vi "Pololu-Convert Degrees to Encoder Units.vi"(4 "Deg Max":u16=180, 5 "Encoder Units Max":u16, 6 "Deg Min":u16, 7 "Encoder Units Min":u16, 8 "Error In":errorcluster, 11 "Position Deg":u16) -> (0 "Error Out":errorcluster, 3 "Position Encoder Units":u16)   [LabVIEW 2018]
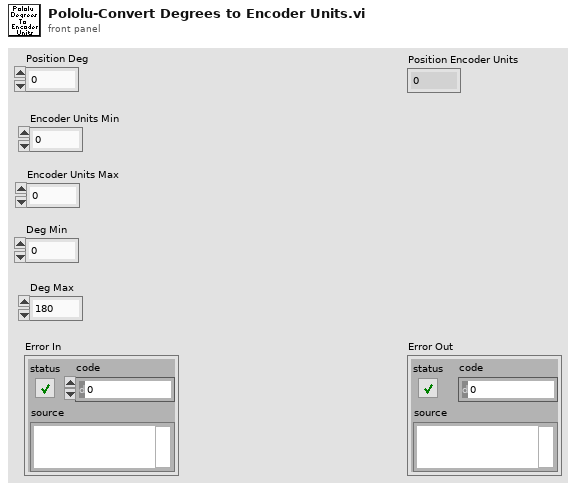
[diagram p1: front panel]
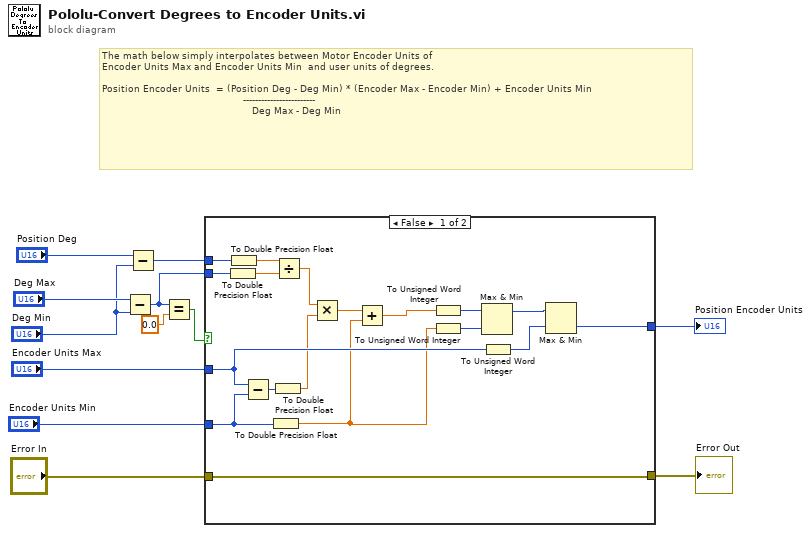
[diagram p0: block diagram]
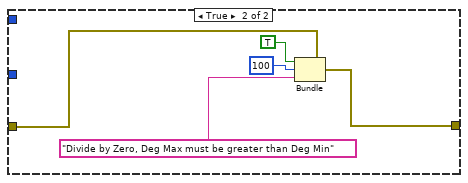
[diagram p2: hidden frame]
diagram:
  # "The math below simply interpolates between Motor Encoder Units of \nEncoder Units Max and Encoder Units Min  and user units of degrees.\n\nPosition Encoder Units  = (Position Deg - Deg Min) * (Encoder Max - Encoder Min) + Encoder Units Min\n                                               ------------------------\n                                                  Deg Max - Deg Min"
  n1 = Subtract(x="Deg Max", y="Deg Min") -> (x-y=w4:u16)
  n2 = Subtract(x="Position Deg", y="Deg Min") -> (x-y=w11:u16)
  n3 = Equal?(x=w4, y=0.0) -> (x = y?=w5:bool)
  n4 = case shown="False" w5 {
    tunnel: [w28 _] -> w12
    tunnel: w11 -> [w20 _]
    tunnel: "Encoder Units Max" -> [w24 _]
    tunnel: "Encoder Units Min" -> [w14 _]
    tunnel: w4 -> [w19 _]
    tunnel: [w21 w31] -> w3
    tunnel: "Error In" -> [w21 w35]
    frame False {
      n5 = To Double Precision Float(number=w19) -> (double precision float=w17:dbl)
      n6 = To Double Precision Float(number=w20) -> (double precision float=w18:dbl)
      n7 = Subtract(x=w24, y=w14) -> (x-y=w16:u16)
      n8 = To Double Precision Float(number=w14) -> (double precision float=w13:dbl)
      n9 = To Double Precision Float(number=w16) -> (double precision float=w15:dbl)
      n10 = Divide(x=w18, y=w17) -> (x/y=w27:dbl)
      n11 = Multiply(x=w27, y=w15) -> (x*y=w23:dbl)
      n12 = Add(x=w23, y=w13) -> (x+y=w22:dbl)
      n13 = To Unsigned Word Integer(number=w22) -> (unsigned 16bit integer=w25:u16)
      n14 = To Unsigned Word Integer(number=w13) -> (unsigned 16bit integer=w26:u16)
      n15 = Max & Min(x=w25, y=w26) -> (max(x,y)=w30:u16)  [unwired: 1 out]
      n16 = To Unsigned Word Integer(number=w24) -> (unsigned 16bit integer=w29:u16)
      n17 = Max & Min(x=w30, y=w29) -> (min(x,y)=w28:u16)  [unwired: 1 out]
    }
    frame True {
      n18 = Bundle(cluster=w35, "status"=TRUE, "code"=100, "source"="Divide by Zero, Deg Max must be greater than Deg Min") -> (w31:errorcluster)
    }
  }
  "Position Encoder Units" <- w12
  "Error Out" <- w3
